vi "st_Percentile Trimming.vi"(10 "p":dbl=25.0, 11 "x array":dbl[](array[numeric])) -> (3 "trimmed x array":dbl[](array[numeric]))   [LabVIEW 2017, in "NI_Gmath.lvlib"]
uses:
  NI_Gmath.lvlib
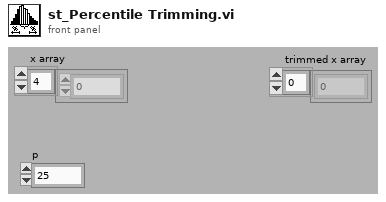
[diagram p1: front panel]
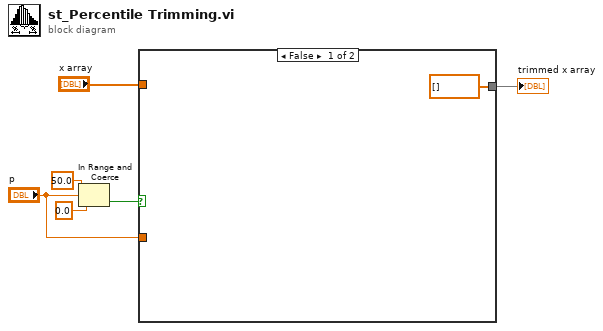
[diagram p0: block diagram]
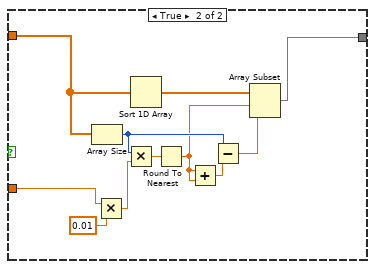
[diagram p2: hidden frame]
diagram:
  n1 = In Range and Coerce(upper limit=50.0, x="p", lower limit=0.0 ("upper limit")) -> (In Range?=w3:bool)  [unwired: 1 out]
  n2 = case shown="False" w3 {
    tunnel: "x array" -> [_ w18]
    tunnel: [dbl[] [] w9] -> w5
    tunnel: "p" -> [_ w8]
    frame False {
    }
    frame True {
      n3 = Array Size(array=w18) -> (size(s)=w13:i32)
      n4 = Multiply(x=w8, y=0.01) -> (x*y=w16:dbl)
      n5 = Multiply(x=w13, y=w16) -> (x*y=w15:dbl)
      n6 = Sort 1D Array(array=w18) -> (sorted array=w14:dbl[])
      n7 = Round To Nearest(number=w15) -> (nearest integer value=w10:dbl)
      n8 = Add(x=w10, y=w10) -> (x+y=w12:dbl)
      n9 = Subtract(x=w13, y=w12) -> (x-y=w11:dbl)
      n10 = Array Subset(array=w14, index=w10, length=w11) -> (w9:dbl[])
    }
  }
  "trimmed x array" <- w5
